vi "test.vi"() -> ()   [LabVIEW 2021, in "Camera.lvlib" / "Camera.lvclass"]
uses:
  Camera/Camera.lvclass
  Camera/Cam task parameters.ctl
  C:/Program Files (x86)/National Instruments/LabVIEW 2021/vi.lib/ActorFramework/Actor/Actor.lvclass
  Camera Messages/Cam prepare task Msg/Cam prepare task Msg.lvclass/Cam prepare task Msg.ctl
  <vilib>/ActorFramework/Message Enqueuer/Message Enqueuer.lvclass/Message Enqueuer.ctl
  <vilib>/ActorFramework/Message Enqueuer/Enqueue.vi
  Camera Messages/Cam prepare task Msg/Cam prepare task Msg.lvclass
  C:/Program Files (x86)/National Instruments/LabVIEW 2021/vi.lib/ActorFramework/Message/Message.lvclass
  Camera Messages/Cam start task Msg/Cam start task Msg.lvclass
  Camera Messages/Cam stop task Msg/Cam stop task Msg.lvclass
  <vilib>/ActorFramework/Stop Msg/Stop Msg.lvclass
  <vilib>/ActorFramework/Message Priority Queue/Priority Enqueue.vi
  <vilib>/ActorFramework/Actor/Actor.lvclass
panel:
  in  "save folder":path
  in  "Cam task parameters":T1
  in  "stop":bool
  in  "start":bool
  in  "prepare":bool
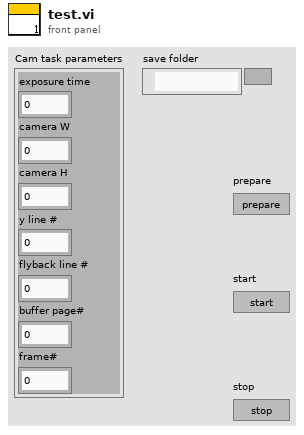
[diagram p1: front panel]
types:
  T1 = typedef "Camera.lvlib/Camera.lvclass/Cam task parameters.ctl" = cluster{"exposure time":dbl, "camera W":dbl, "camera H":dbl, "y line #":dbl, "flyback line #":dbl, "buffer page#":dbl, "frame#":dbl}
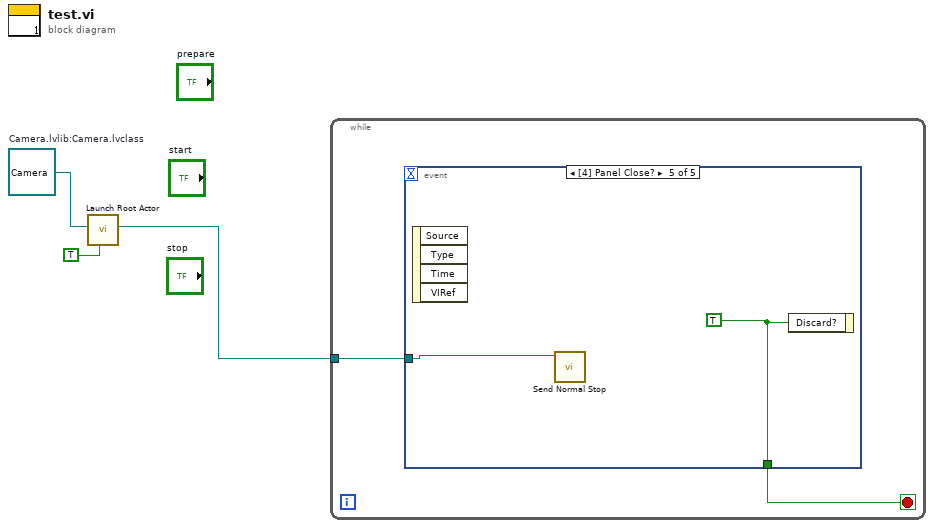
[diagram p0: block diagram]
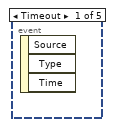
[diagram p2: hidden frame]
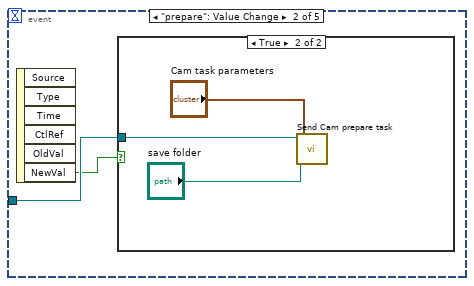
[diagram p3: hidden frame]
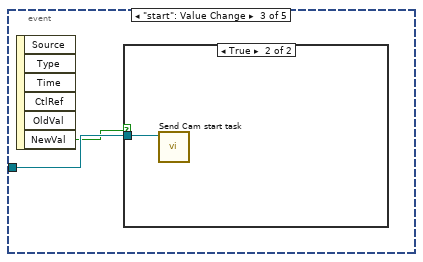
[diagram p5: hidden frame]
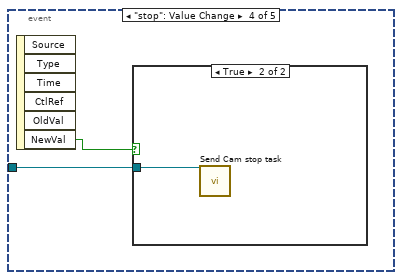
[diagram p7: hidden frame]
diagram:
  w3 = refnum<class "Camera.lvclass"> refnum  # Camera.lvlib:Camera.lvclass
  n1 = call <vilib>:"Launch Root Actor.vi"("Open Actor Core front panel? (F)"=TRUE, "Actor"=w3) -> ("Actor's Enqueuer"=w2:refnum<class "Message Enqueuer.lvclass">)  [unwired: 8 in, 1 out]
  n2 = while {
    tunnel: w2 -> [w4]
    stop <- w5 stop-if-true
    n3 = event shown="[4] Panel Close?" {
      selector: _ -> [_ _ _ _ _]
      dyn-events: _ -> [_ _ _ _ _]
      timeout: _ -> [_ _ _ _ _]
      tunnel: [_ _ _ _ w18] -> w5
      tunnel: w4 -> [_ w7 w12 w15 w17]
      event Timeout {
        n4 = event-data() -> ()  [unwired: 1 in, 3 out]
      }
      event "prepare": Value Change {
        n5 = event-data() -> ("NewVal"=w6:bool)  [unwired: 1 in, 5 out]
        n6 = case shown="True" w6 {
          tunnel: w7 -> [_ w10]
          frame False {
          }
          frame True {
            n7 = call "Send Cam prepare task.vi"("save folder"="save folder", "Cam task parameters"="Cam task parameters", "Message Enqueuer"=w10) -> ()  [unwired: 7 in, 2 out]
          }
        }
      }
      event "start": Value Change {
        n8 = event-data() -> ("NewVal"=w11:bool)  [unwired: 1 in, 5 out]
        n9 = case shown="True" w11 {
          tunnel: w12 -> [_ w13]
          frame False {
          }
          frame True {
            n10 = call "Send Cam start task.vi"("Message Enqueuer"=w13) -> ()  [unwired: 9 in, 2 out]
          }
        }
      }
      event "stop": Value Change {
        n11 = event-data() -> ("NewVal"=w14:bool)  [unwired: 1 in, 5 out]
        n12 = case shown="True" w14 {
          tunnel: w15 -> [_ w16]
          frame False {
          }
          frame True {
            n13 = call "Send Cam stop task.vi"("Message Enqueuer"=w16) -> ()  [unwired: 9 in, 2 out]
          }
        }
      }
      event Panel Close? {
        w18 = TRUE ("Discard?")
        n14 = event-data() -> ()  [unwired: 1 in, 4 out]
        n15 = call <vilib>:"Send Normal Stop.vi"("Message Enqueuer"=w17) -> ()  [unwired: 10 in, 1 out]
        n16 = event-data("Discard?"=w18) -> ()  [unwired: 1 in, 1 out]
      }
    }
  }
